vi "test1.vi"() -> ()   [LabVIEW 2022 SP3]
uses:
  LV_ScreenCapture.dll
  bb1d6301-b892-456f-824b-3fb0d3ec9eb3.vi
panel:
  out "return type":i32
  out "millisecond timer value":u32
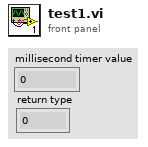
[diagram p1: front panel]
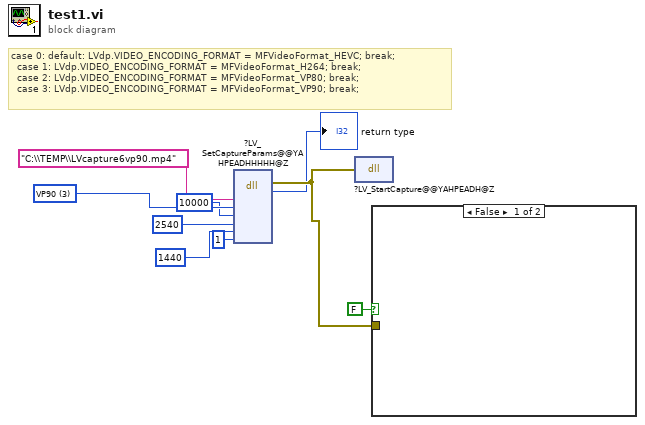
[diagram p0: block diagram]
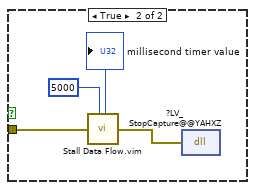
[diagram p2: hidden frame]
diagram:
  w8 = u16 3 items=["HEVC", "H264", "VP80", "VP90"]
  # "case 0: default: LVdp.VIDEO_ENCODING_FORMAT = MFVideoFormat_HEVC; break;\n\t\tcase 1: LVdp.VIDEO_ENCODING_FORMAT = MFVideoFormat_H264; break;\n\t\tcase 2: LVdp.VIDEO_ENCODING_FORMAT = MFVideoFormat_VP80; break;\n\t\tcase 3: LVdp.VIDEO_ENCODING_FORMAT = MFVideoFormat_VP90; break;"
  n1 = dll-call lib="C:/Users/Andrey/Documents/GitHub/ScreenCaptureDirectX/x64/Release/LV_ScreenCapture.dll" fn="?LV_SetCaptureParams@@YAHPEADHHHHH@Z"("path"="C:\\TEMP\\LVcapture6vp90.mp4", "codec"=w8, "duration"=10000, "width"=2540, "height"=1440, "monitor"=1) -> (error out=w6:errorcluster, "return type"=→"return type":i32)  [unwired: 9 in, 1 out]
  n2 = dll-call lib="C:/Users/Andrey/Documents/GitHub/ScreenCaptureDirectX/x64/Release/LV_ScreenCapture.dll" fn="?LV_StartCapture@@YAHPEADH@Z"(error in=w6) -> ()  [unwired: 3 in, 2 out]
  n3 = case shown="False" FALSE {
    tunnel: w6 -> [_ w10]
    frame False {
    }
    frame True {
      n4 = call "Stall Data Flow.vim"("value in"=w10, "milliseconds to wait"=u32 5000) -> ("millisecond timer value"=→"millisecond timer value":u32, "value out"=w12:errorcluster)
      n5 = dll-call lib="C:/Users/Andrey/Documents/GitHub/ScreenCaptureDirectX/x64/Release/LV_ScreenCapture.dll" fn="?LV_StopCapture@@YAHXZ"(error in=w12) -> ()  [unwired: 3 in, 2 out]
    }
  }
